vi "Waveform - Write Waveforms to File.vi"() -> ()   [LabVIEW 2023]
doc: "Shows how to use the Waveform File I/O VIs to write waveform data to a file, and read waveform data from a file."
uses:
  <vilib>/Waveform/WDTFileIO.llb/Write Waveforms to File (1D).vi
  <vilib>/Waveform/WDTFileIO.llb/Export Waveforms To Spreadsheet File (1D).vi
panel:
  out "Waveforms Read from File":waveform(dbl)[](graph)
  out "Waveforms Written to File":waveform(dbl)[](graph)
  # "Overview: Demonstrates the use of the Waveform File I/O VIs to write waveform data to a file, read waveform data from that file, and export waveform data to a spreadsheet file.\nInstructions:\n1. Run this VI. Verify that the waveforms written to the file and read from the file are equal.\n2. Drag the [LabVIEW Data]\\Example Waveform Spreadsheet File.txt file into a spreadsheet application like Microsoft Excel. The data in the file should be automatically populated in the spreadsheet.\n3. Close the spreadsheet application. \n4. Delete the binary file (located at [LabVIEW Data]\\Example Waveform Binary File.dat) and the spreadsheet file (located at [LabVIEW Data]\\Example Waveform Spreadsheet File.txt) when you are done."
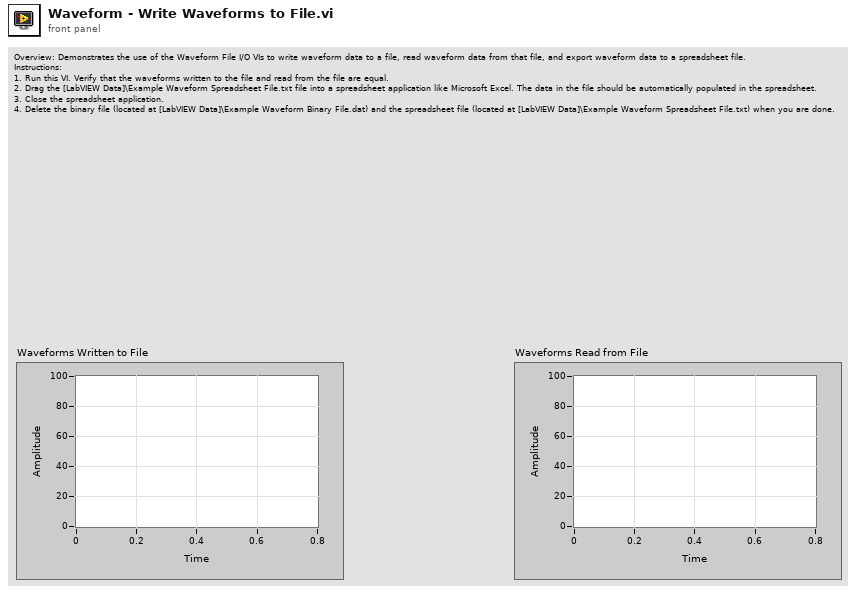
[diagram p1: front panel]
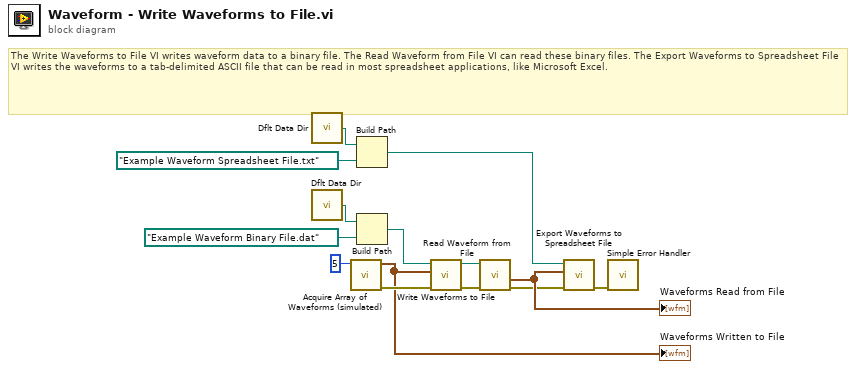
[diagram p0: block diagram]
diagram:
  # "The Write Waveforms to File VI writes waveform data to a binary file. The Read Waveform from File VI can read these binary files. The Export Waveforms to Spreadsheet File VI writes the waveforms to a tab-delimited ASCII file that can be read in most spreadsheet applications, like Microsoft Excel."
  n1 = call <vilib>:"Dflt Data Dir.vi"() -> ("App:Default Data Directory"=w7:path)
  n2 = call <vilib>:"Dflt Data Dir.vi"() -> ("App:Default Data Directory"=w4:path)
  n3 = call "Acquire Array of Waveforms (simulated).vi"("# of waveforms to create"=5) -> ("error out"=w9:errorcluster, "Array of Waveforms"=w1:waveform(dbl)[])  [unwired: 9 in]
  "Waveforms Written to File" <- w1
  n4 = Build Path(base path=w7, name or relative path=path "Example Waveform Spreadsheet File.txt" ("default name")) -> (appended path=w3:path)
  n5 = Build Path(base path=w4, name or relative path=path "Example Waveform Binary File.dat" ("default name")) -> (appended path=w2:path)
  n6 = call-poly <vilib>:"Write Waveforms to File.vi"("error in (no error)"=w9, "waveform array"=w1, "file path (dialog if empty)"=w2) -> ("error out"=w11:errorcluster, "new file path (Not A Path if cancelled)"=w13:path)  [unwired: 7 in]
  n7 = call <vilib>:"Read Waveform from File.vi"("error in (no error)"=w11, "file path (dialog if empty)"=w13) -> ("error out"=w10:errorcluster, "all waveforms in record"=w12:waveform(dbl)[])  [unwired: 4 in, 2 out]
  "Waveforms Read from File" <- w12
  n8 = call-poly <vilib>:"Export Waveforms to Spreadsheet File.vi"("error in (no error)"=w10, "waveforms"=w12, "file path (dialog if empty)"=w3) -> ("error out"=w8:errorcluster)  [unwired: 7 in, 1 out]
  n9 = call <vilib>:"Simple Error Handler.vi"("error in (no error)"=w8) -> ()  [unwired: 4 in, 5 out]
